vi "Re-Anchor steps TreeItemObjs.vi"(10 "indent (i=0)":i32, 11 "TreeItemObjs":refnum<class "BetterItem.lvclass">[](array[class])) -> (3 "TreeItemObjs":refnum<class "BetterItem.lvclass">[](array[class]))   [LabVIEW 2020, in "BetterDragAndDrop.lvlib" / "BetterTreeHandle.lvclass"]
uses:
  BetterTreeHandle/BetterTreeHandle.lvclass
  BetterItem.lvclass
  BetterItem.lvclass/BetterItem.ctl
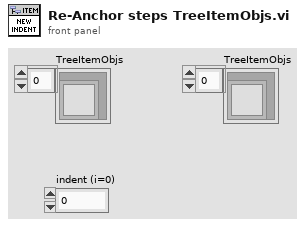
[diagram p1: front panel]
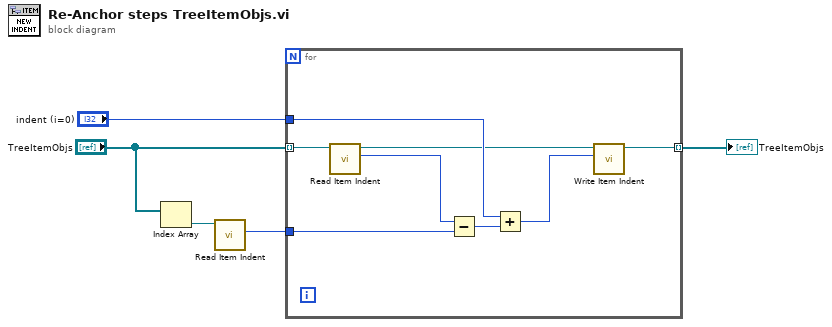
[diagram p0: block diagram]
diagram:
  n1 = Index Array(array="TreeItemObjs") -> (element=w2:refnum<class "BetterItem.lvclass">)  [unwired: 1 in]
  n2 = call "Read Item Indent.vi"("BetterTreeItem in"=w2) -> ("Item Indent"=w1:i32)  [unwired: 9 in, 1 out]
  n3 = for {
    tunnel: "TreeItemObjs" -> [w10] mode=indexing
    tunnel: w1 -> [w13]
    tunnel: "indent (i=0)" -> [w12]
    tunnel: [w7] -> w3 mode=indexing
    n4 = call "Read Item Indent.vi"("BetterTreeItem in"=w10) -> ("Item Indent"=w9:i32, "BetterTreeItem out"=w6:refnum<class "BetterItem.lvclass">)  [unwired: 9 in]
    n5 = Subtract(x=w9, y=w13) -> (x-y=w11:i32)
    n6 = Add(x=w12, y=w11) -> (x+y=w8:i32)
    n7 = call "Write Item Indent.vi"("Item Indent"=w8, "BetterTreeItem in"=w6) -> ("BetterTreeItem out"=w7:refnum<class "BetterItem.lvclass">)  [unwired: 9 in]
  }
  "TreeItemObjs" <- w3
